vi "Enqueue.vi"(7 "Priority Message?":bool, 8 "error in (no error)":errorcluster, 9 "Message Data":variant, 10 "Message":T1, 11 "Message Queue":refnum<queue>) -> (0 "error out":errorcluster, 3 "Message Queue out":refnum<queue>)   [LabVIEW 2024]
uses:
  Message.ctl
  Message Cluster.ctl
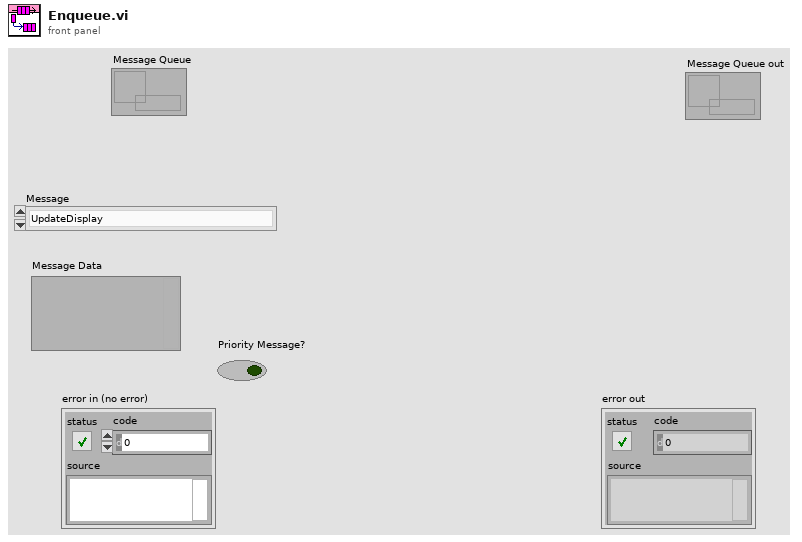
[diagram p1: front panel]
types:
  T1 = typedef "Message.ctl" = enum16{"UpdateDisplay", "Run Washing", "Exit", "Slider run", "Checking wash step", "Continuing washing", "Waiting for slider movement", "Initialize"}
  T2 = typedef "Message Cluster.ctl" = cluster{"Message":T1, "Message Data":variant}
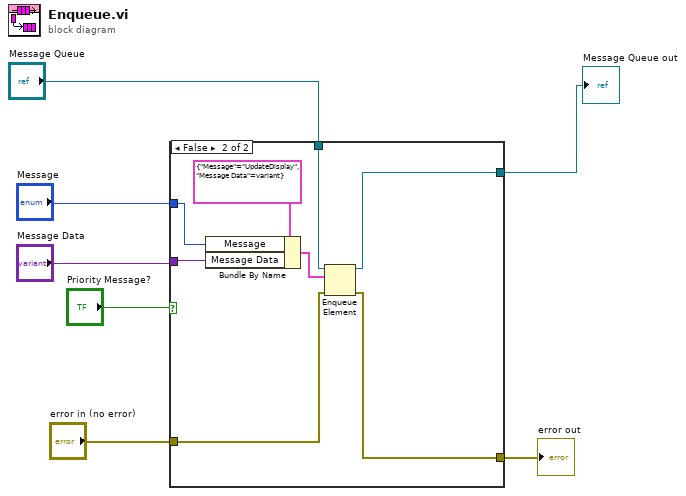
[diagram p0: block diagram]
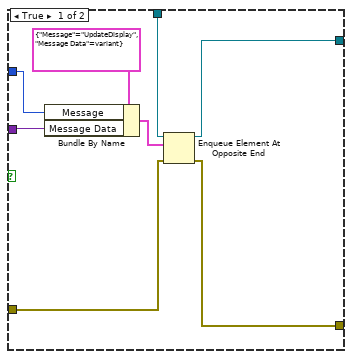
[diagram p2: hidden frame]
diagram:
  n1 = case shown="False" "Priority Message?" {
    tunnel: "Message" -> [w14 w22]
    tunnel: "Message Data" -> [w13 w21]
    tunnel: "error in (no error)" -> [w9 w17]
    tunnel: [w15 w23] -> w2
    tunnel: "Message Queue" -> [w12 w20]
    tunnel: [w8 w16] -> w1
    frame True {
      n2 = Bundle By Name(cluster=T2 {"Message"=enum."UpdateDisplay", "Message Data"=variant} ("Message Cluster 2"), "Message"=w14, "Message Data"=w13) -> (w10:T2)
      n3 = Enqueue Element At Opposite End(queue=w12, element=w10, error in (no error)=w9) -> (queue out=w15:refnum<queue>, error out=w8:errorcluster)  [unwired: 1 in, 1 out]
    }
    frame False {
      n4 = Bundle By Name(cluster=T2 {"Message"=enum."UpdateDisplay", "Message Data"=variant} ("Message Cluster 2"), "Message"=w22, "Message Data"=w21) -> (w18:T2)
      n5 = Enqueue Element(queue=w20, element=w18, error in (no error)=w17) -> (queue out=w23:refnum<queue>, error out=w16:errorcluster)  [unwired: 1 in, 1 out]
    }
  }
  "error out" <- w1
  "Message Queue out" <- w2
